vi "Hardware Scan.vi"(8 "error in (no error)":errorcluster, 11 "Client Controller in":refnum<class "Client Controller.lvclass">) -> (0 "error out":errorcluster, 3 "Client Controller out":refnum<class "Client Controller.lvclass">)   [LabVIEW 2016, in "Client Controller.lvlib" / "Client Controller.lvclass"]
uses:
  Client Controller.lvclass
  C:/Program Files (x86)/National Instruments/LabVIEW 2016/vi.lib/ActorFramework/Actor/Actor.lvclass
  <vilib>/ActorFramework/Actor/Actor.lvclass/Actor.ctl
  <vilib>/ActorFramework/Message Enqueuer/Message Enqueuer.lvclass/Message Enqueuer.ctl
  <vilib>/ActorFramework/Message Enqueuer/Init from Existing Queue.vi
  MAL-Framework/user.lib/Common Components/Controller/Controller.lvclass
  <vilib>/ActorFramework/Message Enqueuer/Message Enqueuer.lvclass
  <vilib>/ActorFramework/Actor/Actor.lvclass
  MAL-Framework/user.lib/Common Components/Controller/Messages/Log Status/Log Status.lvclass
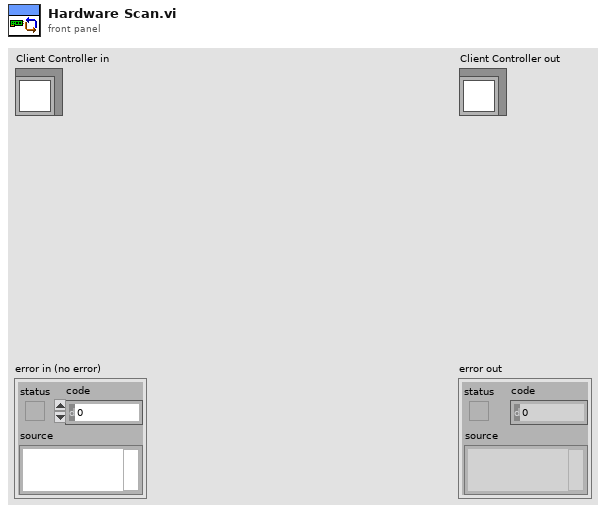
[diagram p1: front panel]
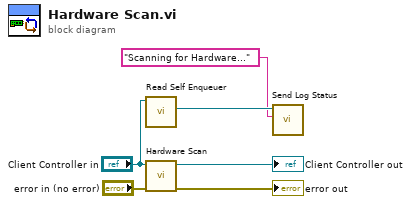
[diagram p0: block diagram]
diagram:
  n1 = call <vilib>:"Read Self Enqueuer.vi"("Actor"="Client Controller in") -> ("Self Enqueuer"=w2:refnum<class "Message Enqueuer.lvclass">)  [unwired: 10 in]
  n2 = call-parent "Hardware Scan.vi"("error in (no error)"="error in (no error)", "Controller in"="Client Controller in") -> ("error out"=→"error out":errorcluster, "Controller out"=→"Client Controller out":refnum<class "Client Controller.lvclass">)  [unwired: 8 in]
  n3 = call "Send Log Status.vi"("String"="Scanning for Hardware...", "Message Enqueuer in"=w2) -> ()  [unwired: 8 in, 2 out]
